vi "set_all_input_names.vi"(8 "error in (no error)":errorcluster, 10 "All input names":string[](array[string]), 11 "VISA resource name":refnum<visa-resource-name>) -> (0 "error out":errorcluster, 3 "VISA resource name out":refnum<visa-resource-name>)   [LabVIEW 2018, in "Inficon IC6.lvlib"]
doc: "Update all input names."
uses:
  <instrlib>/Inficon IC6/Inficon IC6.lvlib
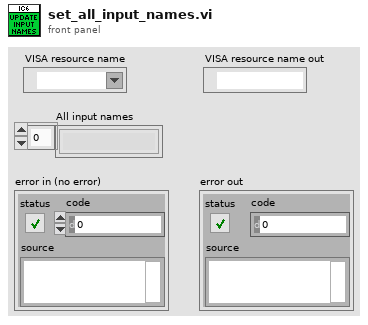
[diagram p1: front panel]
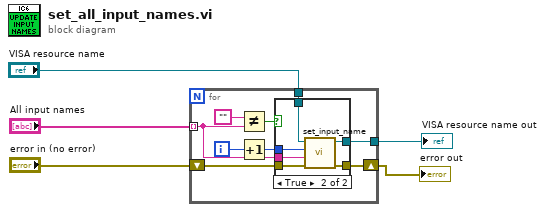
[diagram p0: block diagram]
diagram:
  n1 = for {
    tunnel: "All input names" -> [w10] mode=indexing
    tunnel: "VISA resource name" -> [w9]
    shift-right: [w7] -> w5
    shift-left: "error in (no error)" -> [w8]
    tunnel: [w6] -> w2
    i -> [w14]
    n2 = Not Equal?(x="", y=w10) -> (x != y?=w12:bool)
    n3 = Increment(x=w14) -> (x+1=w13:i32)
    n4 = case shown="True" w12 {
      tunnel: w13 -> [_ w22]
      tunnel: w10 -> [_ w21]
      tunnel: w9 -> [w15 w20]
      tunnel: w8 -> [w16 w19]
      tunnel: [w16 w18] -> w7
      tunnel: [w15 w17] -> w6
      frame False {
      }
      frame True {
        n5 = call <instrlib>:"set_input_name.vi"("error in (no error)"=w19, "input name"=w21, "input number"=w22, "VISA resource name"=w20) -> ("error out"=w18:errorcluster, "VISA resource name out"=w17:refnum<visa-resource-name>)  [unwired: 6 in]
      }
    }
  }
  "error out" <- w5
  "VISA resource name out" <- w2
